vi "Better PID.vi"(1 "Process Variable":dbl, 2 "Setpoint":dbl, 3 "Reset Error Accumulater":bool, 4 "D":dbl format="%.16f", 5 "I":dbl format="%.16f", 6 "P":dbl format="%.16f") -> (0 "Out":dbl)   [LabVIEW 2015]
panel:
  out "Waveform Chart":T1(graph)
  out "Error":dbl
  in  "Error Accumulator":dbl
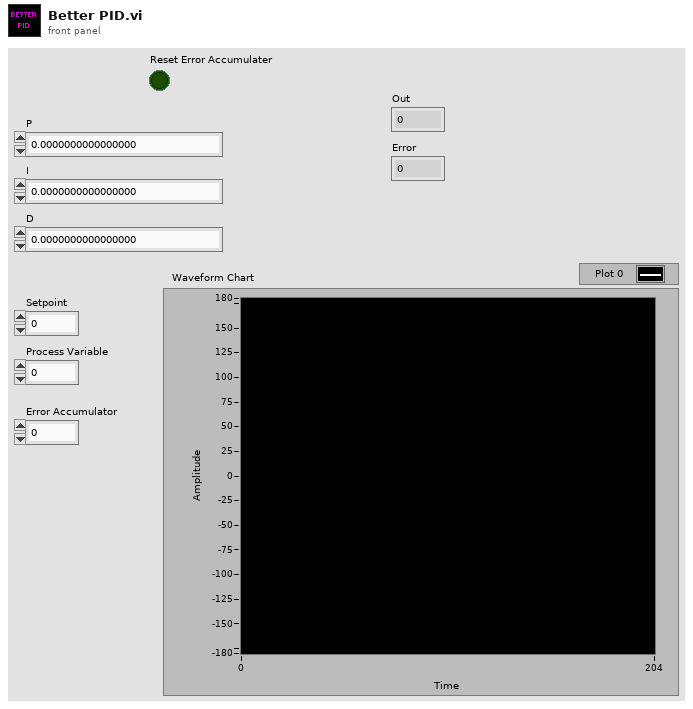
[diagram p1: front panel]
types:
  T1 = cluster{"[0]":dbl, "[1]":dbl, "[2]":dbl, "[3]":dbl, "[4]":dbl, "[5]":dbl, "[6]":dbl, "[7]":dbl, "[8]":dbl}
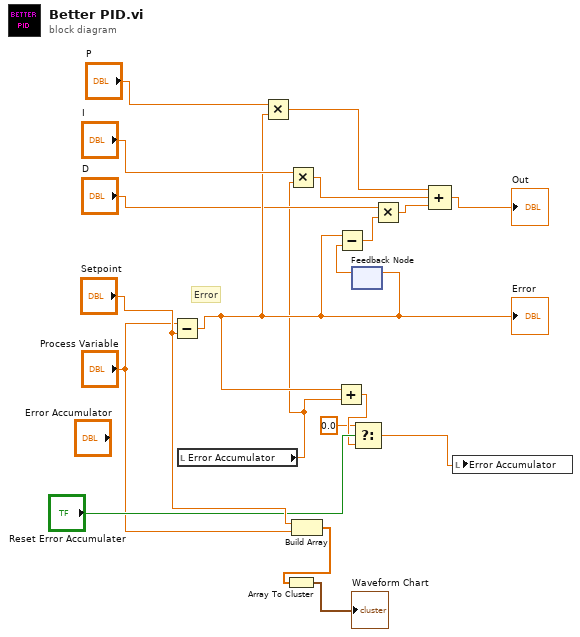
[diagram p0: block diagram]
diagram:
  # "Error"
  n1 = Subtract(x="Process Variable", y="Setpoint") -> (x-y=w15:dbl)
  "Error" <- w15
  n2 = local read "Error Accumulator"() -> (w4:dbl)
  n3 = Multiply(x="P", y=w15) -> (x*y=w18:dbl)
  n4 = Multiply(x="I", y=w4) -> (x*y=w11:dbl)
  n5 = Build Array("Setpoint", "Process Variable") -> (w3:dbl[])
  n6 = Array To Cluster(array=w3) -> (cluster=→"Waveform Chart":T1)
  n7 = Add(x=w15, y=w4) -> (x+y=w7:dbl)
  n8 = feedback-in #1(w15) -> ()
  n9 = feedback #1() -> (w16:dbl)  [unwired: 1 in]
  n10 = Subtract(x=w15, y=w16) -> (x-y=w14:dbl)
  n11 = Select(t=0.0, s="Reset Error Accumulater", f=w7) -> (s? t:f=w6:dbl)
  n12 = Multiply(x="D", y=w14) -> (x*y=w12:dbl)
  n13 = Compound Arithmetic op=ADD(w18, w11, w12) -> (→"Out":dbl)
  n14 = local write "Error Accumulator"(w6) -> ()
